vi "log analysis_gps.vi"() -> ()   [LabVIEW 2018] (continued)
7.8801,22.3000,0.1011,-0.2963,-0.0025,0.185692893,-0.737548130,275.721839304,0.4376,0.2941,0.5694,0.1127,0.0923,0.0781,0.0965,0.1014,4.9971,0f000001,0*33922ff8\n\t", "DUALANTENNAHEADINGA,USB3,0,50.0,FINESTEERING,2107,283447.000,02000000,d426,15824;INSUFFICIENT_OBS,NONE,-1.000000000,0.000000000,0.000000000,0.0,0.000000000,0.000000000,\"631T\",11,4,4,3,04,00,20,03*3318e43a\n\t", "DUALANTENNAHEADINGA,USB3,0,51.5,FINESTEERING,2107,283448.500,02000000,d426,15824;INSUFFICIENT_OBS,NONE,-1.000000000,0.000000000,0.000000000,0.0,0.000000000,0.000000000,\"631T\",14,4,4,3,04,00,20,03*e9e47ab5\n\t", "DUALANTENNAHEADINGA,USB3,0,51.5,FINESTEERING,2107,283449.000,02000000,d426,15824;INSUFFICIENT_OBS,NONE,-1.000000000,0.000000000,0.000000000,0.0,0.000000000,0.000000000,\"631T\",12,4,4,3,04,00,20,03*cef36426\n\t", "DUALANTENNAHEADINGA,USB3,0,49.0,FINESTEERING,2107,283450.000,02000000,d426,15824;INSUFFICIENT_OBS,NONE,-1.000000000,0.000000000,0.000000000,0.0,0.000000000,0.000000000,\"631T\",14,4,4,3,04,00,20,03*09d68f9b\n\t", "DUALANTENNAHEADINGA,USB3,0,49.0,FINESTEERING,2107,283450.500,02000000,d426,15824;INSUFFICIENT_OBS,NONE,-1.000000000,0.000000000,0.000000000,0.0,0.000000000,0.000000000,\"631T\",12,4,4,3,04,00,20,03*431995d1\n\t", "DUALANTENNAHEADINGA,USB3,0,49.0,FINESTEERING,2107,283451.000,02000000,d426,15824;INSUFFICIENT_OBS,NONE,-1.000000000,0.000000000,0.000000000,0.0,0.000000000,0.000000000,\"631T\",12,4,4,3,04,00,20,03*f9d28051\n\t", "DUALANTENNAHEADINGA,USB3,0,44.5,FINESTEERING,2107,283451.500,02000000,d426,15824;INSUFFICIENT_OBS,NONE,-1.000000000,0.000000000,0.000000000,0.0,0.000000000,0.000000000,\"631T\",14,4,4,3,04,00,20,03*5c854f00\n\t", "DUALANTENNAHEADINGA,USB3,0,44.5,FINESTEERING,2107,283452.000,02000000,d426,15824;INSUFFICIENT_OBS,NONE,-1.000000000,0.000000000,0.000000000,0.0,0.000000000,0.000000000,\"631T\",14,4,4,3,04,00,20,03*3dfe5332\n\t", "DUALANTENNAHEADINGA,USB3,0,49.0,FINESTEERING,2107,283452.500,02000000,d426,15824;INSUFFICIENT_OBS,NONE,-1.000000000,0.000000000,0.000000000,0.0,0.000000000,0.000000000,\"631T\",12,4,4,3,04,00,20,03*98a99c63\n\t", "DUALANTENNAHEADINGA,USB3,0,49.0,FINESTEERING,2107,283453.000,02000000,d426,15824;INSUFFICIENT_OBS,NONE,-1.000000000,0.000000000,0.000000000,0.0,0.000000000,0.000000000,\"631T\",10,4,4,3,04,00,20,03*56d68f12\n\t", "DUALANTENNAHEADINGA,USB3,0,50.0,FINESTEERING,2107,283453.500,02000000,d426,15824;INSUFFICIENT_OBS,NONE,-1.000000000,0.000000000,0.000000000,0.0,0.000000000,0.000000000,\"631T\",9,4,4,3,04,00,20,02*71c65a10\n\t", "DUALANTENNAHEADINGA,USB3,0,50.0,FINESTEERING,2107,283454.000,02000000,d426,15824;INSUFFICIENT_OBS,NONE,-1.000000000,0.000000000,0.000000000,0.0,0.000000000,0.000000000,\"631T\",10,4,4,3,04,00,20,03*adf0db7d\n\t", "DUALANTENNAHEADINGA,USB3,0,53.5,FINESTEERING,2107,283454.500,02000000,d426,15824;INSUFFICIENT_OBS,NONE,-1.000000000,0.000000000,0.000000000,0.0,0.000000000,0.000000000,\"631T\",10,4,4,3,04,00,20,03*83545704\n\t", "DUALANTENNAHEADINGA,USB3,0,53.5,FINESTEERING,2107,283455.000,02000000,d426,15824;INSUFFICIENT_OBS,NONE,-1.000000000,0.000000000,0.000000000,0.0,0.000000000,0.000000000,\"631T\",10,4,4,3,04,00,20,03*399f4284\n\t", "DUALANTENNAHEADINGA,USB3,0,53.0,FINESTEERING,2107,283455.500,02000000,d426,15824;INSUFFICIENT_OBS,NONE,-1.000000000,0.000000000,0.000000000,0.0,0.000000000,0.000000000,\"631T\",10,4,4,3,04,00,20,03*bbf6b511\n\t", "DUALANTENNAHEADINGA,USB3,0,53.0,FINESTEERING,2107,283456.000,02000000,d426,15824;INSUFFICIENT_OBS,NONE,-1.000000000,0.000000000,0.000000000,0.0,0.000000000,0.000000000,\"631T\",10,4,4,3,04,00,20,03*da8da923\n\t", "DUALANTENNAHEADINGA,USB3,0,50.5,FINESTEERING,2107,283456.500,02000000,d426,15824;INSUFFICIENT_OBS,NONE,-1.000000000,0.000000000,0.000000000,0.0,0.000000000,0.000000000,\"631T\",10,4,4,3,04,00,20,03*f429255a\n\t", "DUALANTENNAHEADINGA,USB3,0,50.5,FINESTEERING,2107,283457.000,02000000,d426,15824;INSUFFICIENT_OBS,NONE,-1.000000000,0.000000000,0.000000000,0.0,0.000000000,0.000000000,\"631T\",11,4,4,3,04,00,20,03*9900b082\n\t", "DUALANTENNAHEADINGA,USB3,0,52.0,FINESTEERING,2107,283457.500,02000000,d426,15824;INSUFFICIENT_OBS,NONE,-1.000000000,0.000000000,0.000000000,0.0,0.000000000,0.000000000,\"631T\",11,4,4,3,04,00,20,03*d3e0ea5f\n\t", "DUALANTENNAHEADINGA,USB3,0,52.0,FINESTEERING,2107,283458.000,02000000,d426,15824;INSUFFICIENT_OBS,NONE,-1.000000000,0.000000000,0.000000000,0.0,0.000000000,0.000000000,\"631T\",12,4,4,3,04,00,20,02*d2f97f3d\n\t", "INSPVAXA,USB3,0,50.0,FINESTEERING,2107,283458.550,02000000,471d,15824;INS_ALIGNMENT_COMPLETE,INS_RTKFIXED,37.37123761110,126.72265482999,7.8240,22.3000,0.0859,-0.2308,-0.0155,0.304728357,-0.212159203,274.715146909,0.4465,0.2951,0.5711,0.1136,0.0925,0.0781,0.0966,0.1016,5.0109,0f000001,0*14308c9c\n\t", "INSPVAXA,USB3,0,50.0,FINESTEERING,2107,283459.050,02000000,471d,15824;INS_ALIGNMENT_COMPLETE,INS_RTKFIXED,37.37123780985,126.72265328103,7.8227,22.3000,0.0882,-0.3585,-0.0269,0.289946645,-0.080144409,275.013875175,0.4463,0.2950,0.5710,0.1135,0.0925,0.0781,0.0966,0.1016,5.0117,0f000001,0*9875c775\n\t", "INSPVAXA,USB3,0,50.5,FINESTEERING,2107,283459.550,02000000,471d,15824;INS_ALIGNMENT_COMPLETE,INS_RTKFIXED,37.37123799841,126.72265173838,7.8223,22.3000,0.0838,-0.2861,-0.0112,0.173844892,-0.010609871,275.281152331,0.4463,0.2950,0.5710,0.1135,0.0925,0.0781,0.0966,0.1016,5.0117,0f000001,0*d5666360\n\t", "INSPVAXA,USB3,0,50.5,FINESTEERING,2107,283460.050,02000000,471d,15824;INS_ALIGNMENT_COMPLETE,INS_RTKFIXED,37.37123822343,126.72265007400,7.8217,22.3000,0.0923,-0.2835,-0.0262,0.253668906,0.084108634,275.465582577,0.4457,0.2949,0.5709,0.1137,0.0925,0.0781,0.0966,0.1016,5.0129,0f000001,0*4b6161dc\n\t", "INSPVAXA,USB3,0,51.5,FINESTEERING,2107,283460.550,02000000,471d,15824;INS_ALIGNMENT_COMPLETE,INS_RTKFIXED,37.37123844435,126.72264849525,7.8205,22.3000,0.0984,-0.3080,-0.0293,0.364026369,0.239403799,275.671224814,0.4457,0.2949,0.5709,0.1137,0.0925,0.0781,0.0966,0.1016,5.0129,0f000001,0*2bf0cdc4\n\t", "DUALANTENNAHEADINGA,USB3,0,51.5,FINESTEERING,2107,283461.000,02000000,d426,15824;INSUFFICIENT_OBS,NONE,-1.000000000,0.000000000,0.000000000,0.0,0.000000000,0.000000000,\"631T\",13,4,4,3,04,00,20,03*e487ac9d\n\t", "INSPVAXA,USB3,0,47.5,FINESTEERING,2107,283461.550,02000000,471d,15824;INS_ALIGNMENT_COMPLETE,INS_RTKFIXED,37.37123893716,126.72264534248,7.8162,22.3000,0.0985,-0.2963,-0.0141,0.697862948,0.169461107,276.143360178,0.4456,0.2948,0.5708,0.1136,0.0924,0.0781,0.0966,0.1015,5.0137,0f000001,0*a30b3e45\n\t", "INSPVAXA,USB3,0,43.5,FINESTEERING,2107,283462.550,02000000,471d,15824;INS_ALIGNMENT_COMPLETE,INS_RTKFIXED,37.37123942098,126.72264211433,7.8134,22.3000,0.0929,-0.3127,-0.0203,0.398142005,-0.231454144,276.636876132,0.4454,0.2949,0.5708,0.1135,0.0925,0.0781,0.0966,0.1015,5.0146,0f000001,0*24e4ed99\n\t", "INSPVAXA,USB3,0,43.5,FINESTEERING,2107,283463.050,02000000,471d,15824;INS_ALIGNMENT_COMPLETE,INS_RTKFIXED,37.37123965098,126.72264063011,7.8119,22.3000,0.0776,-0.1820,-0.0220,0.127573925,-0.349335206,276.957400381,0.4448,0.2950,0.5707,0.1136,0.0925,0.0781,0.0966,0.1015,5.0158,0f000001,0*86cff0c5\n\t", "INSPVAXA,USB3,0,50.0,FINESTEERING,2107,283463.550,02000000,471d,15824;INS_ALIGNMENT_COMPLETE,INS_RTKFIXED,37.37123983702,126.72263968205,7.8117,22.3000,0.1160,-0.4339,-0.0234,0.042320213,-0.166110227,277.135399170,0.4448,0.2950,0.5707,0.1136,0.0925,0.0781,0.0966,0.1015,5.0158,0f000001,0*a9cde56f\n\t", "INSPVAXA,USB3,0,50.5,FINESTEERING,2107,283464.550,02000000,471d,15824;INS_ALIGNMENT_COMPLETE,INS_RTKFIXED,37.37124035890,126.72263654398,7.8101,22.3000,0.0978,-0.3247,-0.0269,0.153067823,0.062690713,277.456657188,0.4447,0.2949,0.5707,0.1135,0.0925,0.0781,0.0966,0.1015,5.0168,0f000001,0*e25a65bd\n\t", "INSPVAXA,USB3,0,47.5,FINESTEERING,2107,283465.550,02008000,471d,15824;INS_ALIGNMENT_COMPLETE,INS_RTKFIXED,37.37124087816,126.72263323359,7.8095,22.3000,0.1048,-0.3207,-0.0188,-0.139743326,-0.216469066,277.649451326,0.4444,0.2948,0.5707,0.1135,0.0925,0.0781,0.0966,0.1015,5.0179,0f000001,0*3b3a13db\n\t", "INSPVAXA,USB3,0,47.0,FINESTEERING,2107,283466.050,02008000,471d,15824;INS_ALIGNMENT_COMPLETE,INS_RTKFIXED,37.37124115647,126.72263161557,7.8102,22.3000,0.1038,-0.3165,-0.0156,-0.037052070,-0.429278496,277.644852410,0.4437,0.2948,0.5706,0.1136,0.0925,0.0781,0.0966,0.1015,5.0190,0f000001,0*71415a25\n\t", "INSPVAXA,USB3,0,46.5,FINESTEERING,2107,283467.050,02008000,471d,15824;INS_ALIGNMENT_COMPLETE,INS_RTKFIXED,37.37124175185,126.72262828673,7.8114,22.3000,0.1144,-0.3107,-0.0235,0.189502130,-0.846127382,277.724037257,0.4428,0.2947,0.5707,0.1137,0.0925,0.0781,0.0965,0.1015,5.0203,0f000001,0*123a4309\n\t", "INSPVAXA,USB3,0,46.5,FINESTEERING,2107,283467.550,02008000,471d,15824;INS_ALIGNMENT_COMPLETE,INS_RTKFIXED,37.37124201534,126.72262669568,7.8140,22.3000,0.1123,-0.3073,-0.0295,0.009270111,-0.651900427,277.586297393,0.4428,0.2947,0.5707,0.1137,0.0925,0.0781,0.0965,0.1015,5.0203,0f000001,0*fbe18a0e\n\t", "INSPVAXA,USB3,0,46.5,FINESTEERING,2107,283468.050,02008000,471d,15824;INS_ALIGNMENT_COMPLETE,INS_RTKFIXED,37.37124222504,126.72262566051,7.8172,22.3000,0.1108,-0.3362,-0.0087,-0.107061693,-0.300479495,277.280043662,0.4419,0.2947,0.5706,0.1134,0.0926,0.0781,0.0965,0.1015,5.0216,0f000001,0*e4f8bd3b\n\t", "INSPVAXA,USB3,0,46.5,FINESTEERING,2107,283468.550,02008000,471d,15824;INS_ALIGNMENT_COMPLETE,INS_RTKFIXED,37.37124250886,126.72262396333,7.8186,22.3000,0.0904,-0.2606,-0.0155,0.241398611,-0.239914354,276.982575871,0.4419,0.2947,0.5706,0.1134,0.0926,0.0781,0.0965,0.1015,5.0216,0f000001,0*b84fac19\n\t", "INSPVAXA,USB3,0,46.5,FINESTEERING,2107,283469.050,02008000,471d,15824;INS_ALIGNMENT_COMPLETE,INS_RTKFIXED,37.37124277441,126.72262234556,7.8204,22.3000,0.0912,-0.2797,-0.0071,0.371726808,-0.134537847,276.502900110,0.4420,0.2946,0.5707,0.1134,0.0925,0.0781,0.0965,0.1015,5.0228,0f000001,0*e3b85341\n\t", "INSPVAXA,USB3,0,46.5,FINESTEERING,2107,283469.550,02000000,471d,15824;INS_ALIGNMENT_COMPLETE,INS_RTKFIXED,37.37124299469,126.72262074731,7.8238,22.3000,0.0920,-0.2961,-0.0076,0.268432446,-0.051624377,275.936964776,0.4420,0.2946,0.5707,0.1134,0.0925,0.0781,0.0965,0.1015,5.0228,0f000001,0*2bf39c83\n\t", "INSPVAXA,USB3,0,46.5,FINESTEERING,2107,283470.050,02000000,471d,15824;INS_ALIGNMENT_COMPLETE,INS_RTKFIXED,37.37124320185,126.72261913294,7.8277,22.3000,0.1016,-0.3039,-0.0081,0.097334282,-0.040914824,275.470071577,0.4421,0.2945,0.5705,0.1133,0.0925,0.0781,0.0965,0.1015,5.0240,0f000001,0*fba59bc0\n\t", "INSPVAXA,USB3,0,46.0,FINESTEERING,2107,283470.550,02000000,471d,15824;INS_ALIGNMENT_COMPLETE,INS_RTKFIXED,37.37124338791,126.72261753041,7.8308,22.3000,0.0952,-0.3085,-0.0166,0.133198761,-0.149300004,274.919636182,0.4421,0.2945,0.5705,0.1133,0.0925,0.0781,0.0965,0.1015,5.0240,0f000001,0*42261ade\n\t", "INSPVAXA,USB3,0,46.0,FINESTEERING,2107,283471.050,02000000,471d,15824;INS_ALIGNMENT_COMPLETE,INS_RTKFIXED,37.37124356076,126.72261595668,7.8336,22.3000,0.0792,-0.2815,-0.0153,0.105112248,-0.115677362,274.303120166,0.4420,0.2946,0.5706,0.1132,0.0925,0.0781,0.0964,0.1015,5.0248,0f000001,0*c06838c2\n\t", "INSPVAXA,USB3,0,48.0,FINESTEERING,2107,283471.550,02000000,471d,15824;INS_ALIGNMENT_COMPLETE,INS_RTKFIXED,37.37124371844,126.72261435668,7.8362,22.3000,0.0861,-0.3146,0.0012,0.009847777,-0.154362350,273.837649570,0.4420,0.2946,0.5706,0.1132,0.0925,0.0781,0.0964,0.1015,5.0248,0f000001,0*248758d2\n\t", "INSPVAXA,USB3,0,48.0,FINESTEERING,2107,283472.050,02000000,471d,15824;INS_ALIGNMENT_COMPLETE,INS_RTKFIXED,37.37124388873,126.72261272959,7.8390,22.3000,0.0744,-0.3068,0.0071,0.047718600,-0.362449077,273.522239359,0.4416,0.2945,0.5705,0.1131,0.0924,0.0781,0.0964,0.1014,5.0253,0f000001,0*b034cfcb\n\t", "INSPVAXA,USB3,0,48.5,FINESTEERING,2107,283473.050,02000000,471d,15824;INS_ALIGNMENT_COMPLETE,INS_RTKFIXED,37.37124418423,126.72260986099,7.8423,22.3000,0.0465,-0.2147,-0.0152,-0.064754413,-0.661648789,273.035495694,0.4408,0.2944,0.5705,0.1130,0.0925,0.0781,0.0964,0.1014,5.0261,0f000001,0*8452aba9\n\t", "INSPVAXA,USB3,0,49.5,FINESTEERING,2107,283473.550,02000000,471d,15824;INS_ALIGNMENT_COMPLETE,INS_RTKFIXED,37.37124432645,126.72260825595,7.8450,22.3000,0.0577,-0.2717,-0.0116,-0.371304457,-0.586321968,273.022512586,0.4408,0.2944,0.5705,0.1130,0.0925,0.0781,0.0964,0.1014,5.0261,0f000001,0*dc18a2a0\n\t", "INSPVAXA,USB3,0,49.5,FINESTEERING,2107,283474.050,02000000,471d,15824;INS_ALIGNMENT_COMPLETE,INS_RTKFIXED,37.37124450056,126.72260664706,7.8482,22.3000,0.0746,-0.3111,-0.0073,-0.324886266,-0.572903828,273.001550597,0.4404,0.2944,0.5705,0.1132,0.0924,0.0781,0.0964,0.1014,5.0269,0f000001,0*6a9d6035\n\t", "INSPVAXA,USB3,0,47.5,FINESTEERING,2107,283474.550,02000000,471d,15824;INS_ALIGNMENT_COMPLETE,INS_RTKFIXED,37.37124465803,126.72260513334,7.8520,22.3000,0.0754,-0.3176,-0.0107,-0.183521843,-0.419147720,273.001614908,0.4404,0.2944,0.5705,0.1132,0.0924,0.0781,0.0964,0.1014,5.0269,0f000001,0*c3ef68c2\n\t", "INSPVAXA,USB3,0,47.5,FINESTEERING,2107,283475.050,02000000,471d,15824;INS_ALIGNMENT_COMPLETE,INS_RTKFIXED,37.37124482420,126.72260357530,7.8549,22.3000,0.0753,-0.2803,-0.0146,-0.241068696,-0.296923689,273.106112886,0.4399,0.2945,0.5706,0.1130,0.0924,0.0781,0.0964,0.1014,5.0279,0f000001,0*9f37bee3\n\t", "INSPVAXA,USB3,0,47.5,FINESTEERING,2107,283475.550,02000000,471d,15824;INS_ALIGNMENT_COMPLETE,INS_RTKFIXED,37.37124499067,126.72260199547,7.8565,22.3000,0.0685,-0.2996,-0.0135,-0.434680931,-0.247748012,273.252507934,0.4399,0.2945,0.5706,0.1130,0.0924,0.0781,0.0964,0.1014,5.0279,0f000001,0*f6dcb523\n\t", "INSPVAXA,USB3,0,47.5,FINESTEERING,2107,283476.050,02000000,471d,15824;INS_ALIGNMENT_COMPLETE,INS_RTKFIXED,37.37124517702,126.72260043999,7.8594,22.3000,0.0731,-0.2995,-0.0095,-0.441036624,-0.242977977,273.321134070,0.4399,0.2945,0.5707,0.1130,0.0924,0.0781,0.0964,0.1014,5.0290,0f000001,0*df4d40ec\n\t", "INSPVAXA,USB3,0,50.0,FINESTEERING,2107,283476.550,02000000,471d,15824;INS_ALIGNMENT_COMPLETE,INS_RTKFIXED,37.37124535364,126.72259887050,7.8616,22.3000,0.0731,-0.2996,-0.0100,-0.412710306,-0.285107992,273.399842482,0.4399,0.2945,0.5707,0.1130,0.0924,0.0781,0.0964,0.1014,5.0290,0f000001,0*4ef28dbb\n\t", "INSPVAXA,USB3,0,51.0,FINESTEERING,2107,283477.550,02000000,471d,15824;INS_ALIGNMENT_COMPLETE,INS_RTKFIXED,37.37124569782,126.72259576074,7.8655,22.3000,0.0695,-0.3003,-0.0075,-0.469235251,-0.455743841,273.579264680,0.4397,0.2945,0.5707,0.1130,0.0924,0.0781,0.0964,0.1014,5.0303,0f000001,0*db0f6a2f\n\t", "INSPVAXA,USB3,0,51.0,FINESTEERING,2107,283478.050,02000000,471d,15824;INS_ALIGNMENT_COMPLETE,INS_RTKFIXED,37.37124587328,126.72259421546,7.8690,22.3000,0.0786,-0.2811,0.0029,-0.458800403,-0.268524381,273.658587255,0.4407,0.2947,0.5709,0.1132,0.0924,0.0781,0.0964,0.1014,5.0316,0f000001,0*f403e502\n\t", "INSPVAXA,USB3,0,51.0,FINESTEERING,2107,283478.550,02000000,471d,15824;INS_ALIGNMENT_COMPLETE,INS_RTKFIXED,37.37124604525,126.72259266223,7.8723,22.3000,0.0753,-0.2945,0.0030,-0.462352826,-0.136958884,273.744107735,0.4407,0.2947,0.5709,0.1132,0.0924,0.0781,0.0964,0.1014,5.0316,0f000001,0*3bf5fab5\n\t", "INSPVAXA,USB3,0,51.0,FINESTEERING,2107,283479.050,02000000,471d,15824;INS_ALIGNMENT_COMPLETE,INS_RTKFIXED,37.37124622444,126.72259108516,7.8745,22.3000,0.0782,-0.2955,0.0000,-0.529822830,0.178727443,273.870016111,0.4415,0.2947,0.5709,0.1133,0.0924,0.0781,0.0964,0.1014,5.0329,0f000001,0*0db861ca\n\t", "INSPVAXA,USB3,0,51.0,FINESTEERING,2107,283479.550,02000000,471d,15824;INS_ALIGNMENT_COMPLETE,INS_RTKFIXED,37.37124640170,126.72258950006,7.8775,22.3000,0.0805,-0.3037,0.0007,-0.509921072,0.195230583,273.949901234,0.4415,0.2947,0.5709,0.1133,0.0924,0.0781,0.0964,0.1014,5.0329,0f000001,0*077866b6\n\t", "INSPVAXA,USB3,0,51.0,FINESTEERING,2107,283480.050,02000000,471d,15824;INS_ALIGNMENT_COMPLETE,INS_RTKFIXED,37.37124659299,126.72258788570,7.8812,22.3000,0.0832,-0.3022,-0.0023,-0.414591825,-0.152431490,274.036956074,0.4426,0.2949,0.5711,0.1133,0.0924,0.0781,0.0964,0.1014,5.0343,0f000001,0*6e70f737\n\t", "INSPVAXA,USB3,0,50.0,FINESTEERING,2107,283481.550,02000000,471d,15824;INS_ALIGNMENT_COMPLETE,INS_RTKFIXED,37.37124714529,126.72258299767,7.8939,22.3000,0.0873,-0.3069,-0.0133,-0.586135229,-0.604059291,274.319909589,0.4441,0.2951,0.5712,0.1135,0.0925,0.0781,0.0964,0.1015,5.0357,0f000001,0*8645286f\n\t", "INSPVAXA,USB3,0,51.0,FINESTEERING,2107,283482.550,02000000,471d,15824;INS_ALIGNMENT_COMPLETE,INS_RTKFIXED,37.37124752948,126.72258005871,7.9006,22.3000,0.0687,-0.3152,0.0109,-0.135978920,-0.255823048,274.401094363,0.4449,0.2953,0.5713,0.1139,0.0925,0.0782,0.0964,0.1015,5.0373,0f000001,0*5cec8015\n\t", "INSPVAXA,USB3,0,51.5,FINESTEERING,2107,283484.050,02000000,471d,15824;INS_ALIGNMENT_COMPLETE,INS_RTKFIXED,37.37124809880,126.72257534904,7.9142,22.3000,0.0705,-0.2771,0.0043,-0.387988149,0.243310051,274.386615848,0.4464,0.2955,0.5716,0.1138,0.0925,0.0782,0.0964,0.1015,5.0399,0f000001,0*6b4a4f7e\n\t", "INSPVAXA,USB3,0,53.5,FINESTEERING,2107,283485.050,02000000,471d,15824;INS_ALIGNMENT_COMPLETE,INS_RTKFIXED,37.37124849221,126.72257218238,7.9219,22.3000,0.0806,-0.2954,-0.0022,-0.251628518,0.390951997,274.060594650,0.4471,0.2956,0.5717,0.1137,0.0925,0.0782,0.0964,0.1014,5.0410,0f000001,0*78d5c28f\n\t", "INSPVAXA,USB3,0,51.0,FINESTEERING,2107,283485.550,02000000,471d,15824;INS_ALIGNMENT_COMPLETE,INS_RTKFIXED,37.37124867338,126.72257057546,7.9253,22.3000,0.0807,-0.2982,0.0046,-0.297126660,0.143555432,273.789468415,0.4471,0.2956,0.5717,0.1137,0.0925,0.0782,0.0964,0.1014,5.0410,0f000001,0*c848650b\n\t", "INSPVAXA,USB3,0,46.0,FINESTEERING,2107,283486.050,02000000,471d,15824;INS_ALIGNMENT_COMPLETE,INS_RTKFIXED,37.37124886174,126.72256897160,7.9281,22.3000,0.0774,-0.2942,-0.0013,-0.283569757,0.106976902,273.570280777,0.4473,0.2956,0.5718,0.1136,0.0925,0.0782,0.0964,0.1014,5.0421,0f000001,0*a5ad5170\n\t", "INSPVAXA,USB3,0,48.0,FINESTEERING,2107,283487.550,02000000,471d,15824;INS_ALIGNMENT_COMPLETE,INS_RTKFIXED,37.37124935038,126.72256433363,7.9396,22.3000,0.0684,-0.2764,-0.0073,-0.272700392,-0.138830686,272.596264652,0.4472,0.2956,0.5720,0.1137,0.0925,0.0782,0.0964,0.1014,5.0432,0f000001,0*7a2c3ea8\n\t", "INSPVAXA,USB3,0,48.0,FINESTEERING,2107,283488.050,02000000,471d,15824;INS_ALIGNMENT_COMPLETE,INS_RTKFIXED,37.37124950186,126.72256271851,7.9401,22.3000,0.0702,-0.2701,-0.0123,-0.306984619,-0.156481327,272.240352171,0.4472,0.2957,0.5722,0.1136,0.0925,0.0782,0.0964,0.1014,5.0443,0f000001,0*50a165ff\n\t", "INSPVAXA,USB3,0,48.5,FINESTEERING,2107,283488.550,02000000,471d,15824;INS_ALIGNMENT_COMPLETE,INS_RTKFIXED,37.37124963696,126.72256112600,7.9399,22.3000,0.0634,-0.2924,-0.0061,-0.348692985,-0.211479337,271.855613875,0.4472,0.2957,0.5722,0.1136,0.0925,0.0782,0.0964,0.1014,5.0443,0f000001,0*ed71010c\n\t", "INSPVAXA,USB3,0,49.0,FINESTEERING,2107,283489.550,02000000,471d,15824;INS_ALIGNMENT_COMPLETE,INS_RTKFIXED,37.37124992844,126.72255789438,7.9412,22.3000,0.0625,-0.2932,0.0092,-0.217423535,-0.472312164,271.147208708,0.4467,0.2958,0.5722,0.1138,0.0925,0.0782,0.0964,0.1014,5.0457,0f000001,0*6d85d9a8\n\t", "INSPVAXA,USB3,0,49.0,FINESTEERING,2107,283490.050,02000000,471d,15824;INS_ALIGNMENT_COMPLETE,INS_RTKFIXED,37.37125008339,126.72255625341,7.9419,22.3000,0.0636,-0.2955,0.0152,0.008734422,-0.613623948,270.920387351,0.4456,0.2958,0.5721,0.1138,0.0926,0.0782,0.0964,0.1014,5.0473,0f000001,0*aa76f15f\n\t", "INSPVAXA,USB3,0,52.5,FINESTEERING,2107,283490.550,02000000,471d,15824;INS_ALIGNMENT_COMPLETE,INS_RTKFIXED,37.37125019673,126.72255461280,7.9407,22.3000,0.0735,-0.3073,0.0114,-0.028034352,-0.928675652,270.685326293,0.4456,0.2958,0.5721,0.1138,0.0926,0.0782,0.0964,0.1014,5.0473,0f000001,0*cd41eb0e\n\t", "INSPVAXA,USB3,0,49.5,FINESTEERING,2107,283500.050,02000000,471d,15824;INS_ALIGNMENT_COMPLETE,INS_RTKFIXED,37.37125208894,126.72252418884,7.9323,22.3000,0.0457,-0.3130,0.0162,0.019884592,-0.737230354,268.941103131,0.4422,0.2953,0.5719,0.1133,0.0925,0.0782,0.0964,0.1015,5.0570,0f000001,0*24f2188e\n\t", "INSPVAXA,USB3,0,48.5,FINESTEERING,2107,283508.100,02000000,471d,15824;INS_ALIGNMENT_COMPLETE,INS_RTKFIXED,37.37125276901,126.72249960907,7.9453,22.3000,0.0373,-0.2902,0.0053,-0.191217202,-0.027683345,268.229043523,0.4412,0.2949,0.5722,0.1131,0.0925,0.0782,0.0964,0.1013,5.0646,0f000001,0*8b85f82b\n\t", "INSPVAXA,USB3,0,51.0,FINESTEERING,2107,283509.100,02000000,471d,15824;INS_ALIGNMENT_COMPLETE,INS_RTKFIXED,37.37125284410,126.72249644466,7.9470,22.3000,0.0401,-0.2879,-0.0045,-0.106806668,-0.162103067,268.404823616,0.4419,0.2950,0.5723,0.1130,0.0925,0.0782,0.0964,0.1013,5.0643,0f000001,0*7bfc8e45\n\t", "INSPVAXA,USB3,0,49.5,FINESTEERING,2107,283511.100,02000000,471d,15824;INS_ALIGNMENT_COMPLETE,INS_RTKFIXED,37.37125297857,126.72249062368,7.9478,22.3000,0.0268,-0.2671,0.0078,-0.192910717,-0.348782343,268.576521671,0.4435,0.2952,0.5725,0.1132,0.0925,0.0782,0.0964,0.1012,5.0632,0f000001,0*b468220b\n\t", "INSPVAXA,USB3,0,46.5,FINESTEERING,2107,283512.100,02000000,471d,15824;INS_ALIGNMENT_COMPLETE,INS_RTKFIXED,37.37125304820,126.72248734658,7.9477,22.3000,0.0144,-0.2984,0.0121,-0.146751568,-0.096737224,268.816557460,0.4452,0.2954,0.5727,0.1133,0.0925,0.0782,0.0964,0.1013,5.0625,0f000001,0*292499ae\n\t", "INSPVAXA,USB3,0,46.5,FINESTEERING,2107,283512.600,02000000,471d,15824;INS_ALIGNMENT_COMPLETE,INS_RTKFIXED,37.37125307400,126.72248575305,7.9480,22.3000,0.0122,-0.2749,0.0049,-0.358672753,0.036676838,268.917809450,0.4452,0.2954,0.5727,0.1133,0.0925,0.0782,0.0964,0.1013,5.0625,0f000001,0*09269caa\n\t", "INSPVAXA,USB3,0,46.0,FINESTEERING,2107,283516.100,02000000,471d,15824;INS_ALIGNMENT_COMPLETE,INS_RTKFIXED,37.37125347923,126.72247506393,7.9472,22.3000,0.0170,-0.3545,-0.0054,-0.698217493,-0.526151709,269.397858351,0.4451,0.2957,0.5732,0.1136,0.0925,0.0782,0.0963,0.1013,5.0659,0f000001,0*b20fee82\n\t", "INSPVAXA,USB3,0,52.0,FINESTEERING,2107,283517.100,02000000,471d,15824;INS_ALIGNMENT_COMPLETE,INS_RTKFIXED,37.37125363028,126.72247167466,7.9449,22.3000,0.0243,-0.3135,0.0010,-0.686347073,-0.797841284,269.600362862,0.4443,0.2956,0.5732,0.1135,0.0925,0.0782,0.0963,0.1013,5.0669,0f000001,0*80e32c69\n\t", "INSPVAXA,USB3,0,49.0,FINESTEERING,2107,283518.600,02000000,471d,15824;INS_ALIGNMENT_COMPLETE,INS_RTKFIXED,37.37125389857,126.72246679519,7.9445,22.3000,0.0331,-0.3036,0.0138,-0.450567847,-0.447424519,269.738401914,0.4438,0.2956,0.5732,0.1134,0.0925,0.0782,0.0963,0.1013,5.0679,0f000001,0*e0521a7f\n\t", "INSPVAXA,USB3,0,48.0,FINESTEERING,2107,283520.100,02000000,471d,15824;INS_ALIGNMENT_COMPLETE,INS_RTKFIXED,37.37125419691,126.72246226393,7.9458,22.3000,0.0272,-0.1971,0.0083,-0.453121577,-0.197375891,269.782721447,0.4440,0.2956,0.5733,0.1137,0.0925,0.0782,0.0963,0.1013,5.0706,0f000001,0*56a37df9\n\t", "INSPVAXA,USB3,0,51.0,FINESTEERING,2107,283520.600,02000000,471d,15824;INS_ALIGNMENT_COMPLETE,INS_RTKFIXED,37.37125430556,126.72246059927,7.9481,22.3000,0.0288,-0.2781,0.0031,-0.463416060,-0.290924424,269.736679663,0.4440,0.2956,0.5733,0.1137,0.0925,0.0782,0.0963,0.1013,5.0706,0f000001,0*484206e1\n\t", "INSPVAXA,USB3,0,50.0,FINESTEERING,2107,283522.100,02000000,471d,15824;INS_ALIGNMENT_COMPLETE,INS_RTKFIXED,37.37125461142,126.72245575598,7.9554,22.3000,0.0322,-0.2902,-0.0060,-0.575699494,-0.254956238,269.403721782,0.4439,0.2957,0.5734,0.1134,0.0925,0.0782,0.0963,0.1013,5.0736,0f000001,0*4d3ff4ec\n\t", "INSPVAXA,USB3,0,50.0,FINESTEERING,2107,283522.600,02000000,471d,15824;INS_ALIGNMENT_COMPLETE,INS_RTKFIXED,37.37125471396,126.72245415918,7.9561,22.3000,0.0355,-0.2916,-0.0127,-0.527584053,-0.253715800,269.126606548,0.4439,0.2957,0.5734,0.1134,0.0925,0.0782,0.0963,0.1013,5.0736,0f000001,0*ec5fc995\n\t", "INSPVAXA,USB3,0,48.5,FINESTEERING,2107,283523.100,02000000,471d,15824;INS_ALIGNMENT_COMPLETE,INS_RTKFIXED,37.37125482190,126.72245252510,7.9566,22.3000,0.0302,-0.2961,-0.0010,-0.338922460,-0.418464715,268.895183147,0.4433,0.2957,0.5734,0.1134,0.0926,0.0782,0.0963,0.1013,5.0752,0f000001,0*1d6fb429\n\t", "INSPVAXA,USB3,0,48.5,FINESTEERING,2107,283523.600,02000000,471d,15824;INS_ALIGNMENT_COMPLETE,INS_RTKFIXED,37.37125490537,126.72245090226,7.9573,22.3000,0.0299,-0.3022,0.0033,-0.516635552,-0.400593547,268.699996239,0.4433,0.2957,0.5734,0.1134,0.0926,0.0782,0.0963,0.1013,5.0752,0f000001,0*027b4151\n\t", "INSPVAXA,USB3,0,49.5,FINESTEERING,2107,283524.100,02000000,471d,15824;INS_ALIGNMENT_COMPLETE,INS_RTKFIXED,37.37125498193,126.72244929891,7.9584,22.3000,0.0403,-0.2922,0.0032,-0.646627486,-0.365479151,268.410156940,0.4428,0.2959,0.5733,0.1133,0.0925,0.0782,0.0963,0.1013,5.0766,0f000001,0*7811970f\n\t", "INSPVAXA,USB3,0,47.5,FINESTEERING,2107,283525.600,02000000,471d,15824;INS_ALIGNMENT_COMPLETE,INS_RTKFIXED,37.37125519906,126.72244452104,7.9610,22.3000,0.0264,-0.2896,0.0115,-0.459568698,-0.292533166,267.670803857,0.4424,0.2958,0.5732,0.1133,0.0925,0.0782,0.0963,0.1013,5.0781,0f000001,0*17724b4e\n\t", "INSPVAXA,USB3,0,47.0,FINESTEERING,2107,283526.100,02008000,471d,15824;INS_ALIGNMENT_COMPLETE,INS_RTKFIXED,37.37125524446,126.72244292133,7.9621,22.3000,0.0343,-0.2757,0.0102,-0.752609295,-0.423876797,267.522844293,0.4423,0.2959,0.5731,0.1133,0.0925,0.0782,0.0963,0.1013,5.0795,0f000001,0*e02a1c85\n\t", "INSPVAXA,USB3,0,47.0,FINESTEERING,2107,283527.100,02008000,471d,15824;INS_ALIGNMENT_COMPLETE,INS_RTKFIXED,37.37125535577,126.72243973319,7.9657,22.3000,0.0385,-0.2807,-0.0002,-0.916031014,-0.466994988,267.419817945,0.4418,0.2957,0.5731,0.1132,0.0925,0.0782,0.0963,0.1013,5.0811,0f000001,0*de1342cb\n\t", "INSPVAXA,USB3,0,48.0,FINESTEERING,2107,283527.600,02008000,471d,15824;INS_ALIGNMENT_COMPLETE,INS_RTKFIXED,37.37125539878,126.72243810634,7.9658,22.3000,0.0326,-0.2757,-0.0036,-1.071635503,-0.660283197,267.417863682,0.4418,0.2957,0.5731,0.1132,0.0925,0.0782,0.0963,0.1013,5.0811,0f000001,0*715093d1\n\t", "INSPVAXA,USB3,0,46.5,FINESTEERING,2107,283528.100,02008000,471d,15824;INS_ALIGNMENT_COMPLETE,INS_RTKFIXED,37.37125544077,126.72243647488,7.9658,22.3000,0.0284,-0.2919,-0.0061,-1.262244823,-0.886371740,267.477769914,0.4412,0.2955,0.5730,0.1131,0.0925,0.0782,0.0963,0.1013,5.0826,0f000001,0*a5d2d267\n\t", "INSPVAXA,USB3,0,51.5,FINESTEERING,2107,283529.100,02008000,471d,15824;INS_ALIGNMENT_COMPLETE,INS_RTKFIXED,37.37125551038,126.72243332814,7.9661,22.3000,0.0230,-0.2496,0.0003,-1.593217414,-1.364879356,267.511520433,0.4406,0.2953,0.5729,0.1132,0.0926,0.0782,0.0963,0.1012,5.0841,0f000001,0*c5d25f23\n\t", "INSPVAXA,USB3,0,51.5,FINESTEERING,2107,283529.600,02008000,471d,15824;INS_ALIGNMENT_COMPLETE,INS_RTKFIXED,37.37125553545,126.72243179074,7.9678,22.3000,0.0177,-0.3268,0.0196,-1.900322132,-1.296600351,267.646844528,0.4406,0.2953,0.5729,0.1132,0.0926,0.0782,0.0963,0.1012,5.0841,0f000001,0*bf0a8b51\n\t", "INSPVAXA,USB3,0,51.0,FINESTEERING,2107,283530.100,02008000,471d,15824;INS_ALIGNMENT_COMPLETE,INS_RTKFIXED,37.37125556979,126.72243022543,7.9689,22.3000,0.0347,-0.2712,0.0165,-2.106253221,-1.191638715,267.711415615,0.4397,0.2950,0.5729,0.1130,0.0929,0.0782,0.0963,0.1012,5.0852,0f000001,0*30fd5459\n\t", "INSPVAXA,USB3,0,51.0,FINESTEERING,2107,283530.600,02000000,471d,15824;INS_ALIGNMENT_COMPLETE,INS_RTKFIXED,37.37125561825,126.72242855799,7.9691,22.3000,0.0407,-0.2688,0.0120,-2.213736166,-1.038882938,267.844151397,0.4397,0.2950,0.5729,0.1130,0.0929,0.0782,0.0963,0.1012,5.0852,0f000001,0*ed713259\n\t", "INSPVAXA,USB3,0,43.5,FINESTEERING,2107,283531.100,02000000,471d,15824;INS_ALIGNMENT_COMPLETE,INS_RTKFIXED,37.37125567803,126.72242699713,7.9701,22.3000,0.0384,-0.2967,0.0169,-2.258821559,-0.728124735,267.962573337,0.4398,0.2947,0.5728,0.1130,0.0928,0.0782,0.0963,0.1012,5.0855,0f000001,0*96bde39a\n\t", "INSPVAXA,USB3,0,43.5,FINESTEERING,2107,283531.600,02000000,471d,15824;INS_ALIGNMENT_COMPLETE,INS_RTKFIXED,37.37125573053,126.72242543109,7.9712,22.3000,0.0393,-0.2946,0.0161,-2.393557008,-0.508805819,268.092577363,0.4398,0.2947,0.5728,0.1130,0.0928,0.0782,0.0963,0.1012,5.0855,0f000001,0*fb176aea\n\t", "INSPVAXA,USB3,0,46.5,FINESTEERING,2107,283532.600,02000000,471d,15824;INS_ALIGNMENT_COMPLETE,INS_RTKFIXED,37.37125585668,126.72242215627,7.9725,22.3000,0.0380,-0.3002,0.0167,-2.444436463,-0.411927002,268.408506598,0.4408,0.2948,0.5728,0.1133,0.0928,0.0782,0.0963,0.1013,5.0851,0f000001,0*752f38e5\n\t", "INSPVAXA,USB3,0,46.5,FINESTEERING,2107,283533.100,02000000,471d,15824;INS_ALIGNMENT_COMPLETE,INS_RTKFIXED,37.37125592571,126.72242055610,7.9738,22.3000,0.0424,-0.2920,0.0172,-2.420399044,-0.549310631,268.532317727,0.4414,0.2948,0.5728,0.1132,0.0926,0.0782,0.0963,0.1012,5.0840,0f000001,0*330bd1f6\n\t", "INSPVAXA,USB3,0,49.5,FINESTEERING,2107,283533.600,02000000,471d,15824;INS_ALIGNMENT_COMPLETE,INS_RTKFIXED,37.37125599617,126.72241909319,7.9758,22.3000,0.0239,-0.2932,0.0057,-2.389135000,-0.690009705,268.630043000,0.4414,0.2948,0.5728,0.1132,0.0926,0.0782,0.0963,0.1012,5.0840,0f000001,0*946e4f45\n\t", "INSPVAXA,USB3,0,46.5,FINESTEERING,2107,283534.100,02000000,471d,15824;INS_ALIGNMENT_COMPLETE,INS_RTKFIXED,37.37125606459,126.72241729161,7.9768,22.3000,0.0318,-0.3014,0.0051,-2.433419723,-0.928712698,268.813892776,0.4412,0.2949,0.5728,0.1131,0.0925,0.0782,0.0963,0.1012,5.0833,0f000001,0*8f6d80c9\n\t", "INSPVAXA,USB3,0,46.5,FINESTEERING,2107,283534.600,02000000,471d,15824;INS_ALIGNMENT_COMPLETE,INS_RTKFIXED,37.37125615079,126.72241575292,7.9767,22.3000,0.0422,-0.2723,0.0071,-2.318351029,-0.994572866,268.928791382,0.4412,0.2949,0.5728,0.1131,0.0925,0.0782,0.0963,0.1012,5.0833,0f000001,0*09e2fdbf\n\t", "INSPVAXA,USB3,0,46.5,FINESTEERING,2107,283535.100,02000000,471d,15824;INS_ALIGNMENT_COMPLETE,INS_RTKFIXED,37.37125625866,126.72241406717,7.9767,22.3000,0.0424,-0.2966,-0.0053,-2.021295828,-1.106669357,269.086555595,0.4405,0.2950,0.5729,0.1131,0.0926,0.0782,0.0963,0.1012,5.0840,0f000001,0*6efa0b45\n\t", "INSPVAXA,USB3,0,46.5,FINESTEERING,2107,283535.600,02000000,471d,15824;INS_ALIGNMENT_COMPLETE,INS_RTKFIXED,37.37125636363,126.72241247006,7.9775,22.3000,0.0475,-0.2765,0.0068,-1.865554802,-1.007723760,269.206912297,0.4405,0.2950,0.5729,0.1131,0.0926,0.0782,0.0963,0.1012,5.0840,0f000001,0*0c6af5d6\n\t", "INSPVAXA,USB3,0,47.5,FINESTEERING,2107,283536.100,02000000,471d,15824;INS_ALIGNMENT_COMPLETE,INS_RTKFIXED,37.37125647369,126.72241083113,7.9788,22.3000,0.0521,-0.3007,0.0049,-1.790943231,-0.806222731,269.320889615,0.4398,0.2953,0.5729,0.1129,0.0928,0.0782,0.0963,0.1012,5.0856,0f000001,0*d4e8effb\n\t", "INSPVAXA,USB3,0,47.5,FINESTEERING,2107,283536.600,02000000,471d,15824;INS_ALIGNMENT_COMPLETE,INS_RTKFIXED,37.37125658130,126.72240921238,7.9784,22.3000,0.0588,-0.2967,0.0032,-1.856879731,-0.578836067,269.400871435,0.4398,0.2953,0.5729,0.1129,0.0928,0.0782,0.0963,0.1012,5.0856,0f000001,0*690b56d4\n\t", "INSPVAXA,USB3,0,46.0,FINESTEERING,2107,283537.100,02000000,471d,15824;INS_ALIGNMENT_COMPLETE,INS_RTKFIXED,37.37125671293,126.72240759051,7.9784,22.3000,0.0622,-0.2885,0.0100,-1.691821646,-0.334147317,269.491731881,0.4392,0.2956,0.5729,0.1129,0.0929,0.0782,0.0963,0.1012,5.0866,0f000001,0*9d354d84\n\t", "INSPVAXA,USB3,0,46.0,FINESTEERING,2107,283537.600,02000000,471d,15824;INS_ALIGNMENT_COMPLETE,INS_RTKFIXED,37.37125683698,126.72240594411,7.9786,22.3000,0.0572,-0.2873,0.0166,-1.418143186,-0.126899320,269.581521554,0.4392,0.2956,0.5729,0.1129,0.0929,0.0782,0.0963,0.1012,5.0866,0f000001,0*6d004f4c\n\t", "INSPVAXA,USB3,0,49.0,FINESTEERING,2107,283538.100,02000000,471d,15824;INS_ALIGNMENT_COMPLETE,INS_RTKFIXED,37.37125695995,126.72240477426,7.9799,22.3000,0.0495,-0.1342,0.0227,-1.319474925,-0.166358731,269.556076061,0.4404,0.2961,0.5730,0.1144,0.0933,0.0783,0.0963,0.1012,5.0866,0f000001,0*5c5cf594\n\t", "INSPVAXA,USB3,0,49.0,FINESTEERING,2107,283538.600,02000000,471d,15824;INS_ALIGNMENT_COMPLETE,INS_RTKFIXED,37.37125706097,126.72240298813,7.9830,22.3000,0.0438,-0.2893,0.0273,-1.369512709,-0.160060416,269.600478230,0.4404,0.2961,0.5730,0.1144,0.0933,0.0783,0.0963,0.1012,5.0866,0f000001,0*64f2f597\n\t", "INSPVAXA,USB3,0,51.0,FINESTEERING,2107,283539.100,02000000,471d,15824;INS_ALIGNMENT_COMPLETE,INS_RTKFIXED,37.37125716893,126.72240151116,7.9851,22.3000,0.0349,-0.3370,0.0409,-1.494089497,0.116619175,269.541070998,0.4422,0.2966,0.5733,0.1130,0.0931,0.0783,0.0963,0.1012,5.0845,0f000001,0*15f1df55\n\t", "INSPVAXA,USB3,0,51.0,FINESTEERING,2107,283539.600,02000000,471d,15824;INS_ALIGNMENT_COMPLETE,INS_RTKFIXED,37.37125727133,126.72239988665,7.9877,22.3000,0.0429,-0.2928,0.0329,-1.461817471,0.138335830,269.463131487,0.4422,0.2966,0.5733,0.1130,0.0931,0.0783,0.0963,0.1012,5.0845,0f000001,0*8c571713\n\t", "INSPVAXA,USB3,0,50.0,FINESTEERING,2107,283540.100,02000000,471d,15824;INS_ALIGNMENT_COMPLETE,INS_RTKFIXED,37.37125737761,126.72239824656,7.9900,22.3000,0.0519,-0.2782,0.0221,-1.451094613,0.074238516,269.298675528,0.4419,0.2969,0.5734,0.1130,0.0929,0.0783,0.0963,0.1012,5.0817,0f000001,0*b323d296\n\t", "INSPVAXA,USB3,0,50.0,FINESTEERING,2107,283540.600,02000000,471d,15824;INS_ALIGNMENT_COMPLETE,INS_RTKFIXED,37.37125746759,126.72239663487,7.9912,22.3000,0.0429,-0.2872,0.0160,-1.425165250,-0.019252695,269.086348976,0.4419,0.2969,0.5734,0.1130,0.0929,0.0783,0.0963,0.1012,5.0817,0f000001,0*88d26abe\n\t", "INSPVAXA,USB3,0,47.0,FINESTEERING,2107,283541.100,02000000,471d,15824;INS_ALIGNMENT_COMPLETE,INS_RTKFIXED,37.37125754334,126.72239500157,7.9927,22.3000,0.0440,-0.2830,0.0173,-1.652300860,-0.379493530,268.915877089,0.4417,0.2969,0.5736,0.1129,0.0927,0.0783,0.0963,0.1011,5.0789,0f000001,0*58806b1d\n\t", "INSPVAXA,USB3,0,47.0,FINESTEERING,2107,283541.600,02000000,471d,15824;INS_ALIGNMENT_COMPLETE,INS_RTKFIXED,37.37125761933,126.72239337708,7.9953,22.3000,0.0493,-0.2834,0.0162,-1.785773716,-0.511638678,268.665930676,0.4417,0.2969,0.5736,0.1129,0.0927,0.0783,0.0963,0.1011,5.0789,0f000001,0*bd9c5353\n\t", "INSPVAXA,USB3,0,48.5,FINESTEERING,2107,283542.100,02000000,471d,15824;INS_ALIGNMENT_COMPLETE,INS_RTKFIXED,37.37125769665,126.72239177679,7.9980,22.3000,0.0493,-0.2951,0.0235,-1.875048061,-0.540533252,268.386297576,0.4405,0.2966,0.5735,0.1128,0.0925,0.0783,0.0963,0.1011,5.0773,0f000001,0*2be40074\n\t", "INSPVAXA,USB3,0,48.5,FINESTEERING,2107,283542.600,02000000,471d,15824;INS_ALIGNMENT_COMPLETE,INS_RTKFIXED,37.37125775872,126.72239016301,7.9996,22.3000,0.0518,-0.3025,0.0218,-1.945640979,-0.365484318,268.174264778,0.4405,0.2966,0.5735,0.1128,0.0925,0.0783,0.0963,0.1011,5.0773,0f000001,0*896be2ff\n\t", "INSPVAXA,USB3,0,47.5,FINESTEERING,2107,283543.100,02000000,471d,15824;INS_ALIGNMENT_COMPLETE,INS_RTKFIXED,37.37125783022,126.72238854441,8.0007,22.3000,0.0360,-0.2808,0.0229,-1.906190638,-0.356725874,267.886535177,0.4398,0.2962,0.5735,0.1128,0.0925,0.0783,0.0963,0.1011,5.0772,0f000001,0*1744d296\n\t", "INSPVAXA,USB3,0,47.5,FINESTEERING,2107,283543.600,02000000,471d,15824;INS_ALIGNMENT_COMPLETE,INS_RTKFIXED,37.37125788763,126.72238692132,8.0016,22.3000,0.0356,-0.2896,0.0094,-1.979603347,-0.321373170,267.681718152,0.4398,0.2962,0.5735,0.1128,0.0925,0.0783,0.0963,0.1011,5.0772,0f000001,0*45f837fc\n\t", "DUALANTENNAHEADINGA,USB3,0,47.5,FINESTEERING,2107,283544.100,02000000,d426,15824;INSUFFICIENT_OBS,NONE,-1.000000000,0.000000000,0.000000000,0.0,0.000000000,0.000000000,\"631T\",12,4,4,3,04,00,20,02*84d96ce8\n\t", "INSPVAXA,USB3,0,51.0,FINESTEERING,2107,283544.600,02000000,471d,15824;INS_ALIGNMENT_COMPLETE,INS_RTKFIXED,37.37125797814,126.72238366933,8.0025,22.3000,0.0382,-0.2769,0.0143,-2.206615640,-0.357729210,267.363519498,0.4396,0.2961,0.5737,0.1128,0.0924,0.0783,0.0964,0.1011,5.0776,0f000001,0*0a578cde\n\t", "INSPVAXA,USB3,0,49.5,FINESTEERING,2107,283545.100,02000000,471d,15824;INS_ALIGNMENT_COMPLETE,INS_RTKFIXED,37.37125803132,126.72238203676,8.0019,22.3000,0.0517,-0.2764,0.0124,-2.158934023,-0.436592254,267.230007610,0.4389,0.2957,0.5737,0.1127,0.0924,0.0783,0.0964,0.1011,5.0787,0f000001,0*62787010\n\t", "INSPVAXA,USB3,0,49.5,FINESTEERING,2107,283545.600,02000000,471d,15824;INS_ALIGNMENT_COMPLETE,INS_RTKFIXED,37.37125808188,126.72238043700,8.0001,22.3000,0.0477,-0.2875,0.0096,-2.125628520,-0.371940065,267.210451376,0.4389,0.2957,0.5737,0.1127,0.0924,0.0783,0.0964,0.1011,5.0787,0f000001,0*6d8598a7\n\t", "DUALANTENNAHEADINGA,USB3,0,49.0,FINESTEERING,2107,283546.100,02000000,d426,15824;INSUFFICIENT_OBS,NONE,-1.000000000,0.000000000,0.000000000,0.0,0.000000000,0.000000000,\"631T\",14,4,4,3,04,00,20,03*f6e7f028\n\t", "INSPVAXA,USB3,0,49.0,FINESTEERING,2107,283546.600,02000000,471d,15824;INS_ALIGNMENT_COMPLETE,INS_RTKFIXED,37.37125815693,126.72237718708,7.9959,22.3000,0.0472,-0.2869,0.0097,-2.448876962,-0.301078601,267.272161666,0.4388,0.2955,0.5737,0.1127,0.0924,0.0783,0.0964,0.1011,5.0802,0f000001,0*b5ddd59b\n\t", "DUALANTENNAHEADINGA,USB3,0,49.0,FINESTEERING,2107,283547.100,02000000,d426,15824;INSUFFICIENT_OBS,NONE,-1.000000000,0.000000000,0.000000000,0.0,0.000000000,0.000000000,\"631T\",13,4,4,3,04,00,20,03*d1017fba\n\t", "DUALANTENNAHEADINGA,USB3,0,50.5,FINESTEERING,2107,283547.600,02000000,d426,15824;INSUFFICIENT_OBS,NONE,-1.000000000,0.000000000,0.000000000,0.0,0.000000000,0.000000000,\"631T\",14,4,4,3,04,00,20,03*23b2448a\n\t", "INSPVAXA,USB3,0,48.5,FINESTEERING,2107,283548.100,02000000,471d,15824;INS_ALIGNMENT_COMPLETE,INS_RTKFIXED,37.37125826747,126.72237261641,7.9908,22.3000,0.0551,-0.2062,0.0107,-2.709225073,-0.117327049,267.249046746,0.4386,0.2951,0.5737,0.1130,0.0926,0.0783,0.0964,0.1011,5.0831,0f000001,0*59a87063\n\t", "INSPVAXA,USB3,0,48.5,FINESTEERING,2107,283548.600,02000000,471d,15824;INS_ALIGNMENT_COMPLETE,INS_RTKFIXED,37.37125828182,126.72237093999,7.9873,22.3000,0.0467,-0.3123,0.0115,-2.842538161,-0.073425539,267.267184569,0.4386,0.2951,0.5737,0.1130,0.0926,0.0783,0.0964,0.1011,5.0831,0f000001,0*3db09e30\n\t", "INSPVAXA,USB3,0,49.0,FINESTEERING,2107,283549.100,02000000,471d,15824;INS_ALIGNMENT_COMPLETE,INS_RTKFIXED,37.37125831392,126.72236948257,7.9859,22.3000,0.0458,-0.3107,0.0117,-2.935659020,0.110600359,267.341322191,0.4389,0.2949,0.5737,0.1127,0.0927,0.0783,0.0964,0.1010,5.0837,0f000001,0*651f733f\n\t", "DUALANTENNAHEADINGA,USB3,0,49.0,FINESTEERING,2107,283549.600,02000000,d426,15824;INSUFFICIENT_OBS,NONE,-1.000000000,0.000000000,0.000000000,0.0,0.000000000,0.000000000,\"631T\",12,4,4,3,04,00,20,03*a5c8d3a9\n\t", "INSPVAXA,USB3,0,49.0,FINESTEERING,2107,283550.100,02000000,471d,15824;INS_ALIGNMENT_COMPLETE,INS_RTKFIXED,37.37125837980,126.72236622244,7.9865,22.3000,0.0464,-0.2979,0.0062,-2.970555166,0.308033741,267.553888887,0.4387,0.2947,0.5737,0.1126,0.0926,0.0783,0.0963,0.1010,5.0837,0f000001,0*d140be5a\n\t", "INSPVAXA,USB3,0,50.5,FINESTEERING,2107,283550.600,02000000,471d,15824;INS_ALIGNMENT_COMPLETE,INS_RTKFIXED,37.37125841199,126.72236465933,7.9851,22.3000,0.0388,-0.2917,0.0030,-2.826015531,0.302597414,267.642559027,0.4387,0.2947,0.5737,0.1126,0.0926,0.0783,0.0963,0.1010,5.0837,0f000001,0*d1068808\n\t", "DUALANTENNAHEADINGA,USB3,0,46.5,FINESTEERING,2107,283551.100,02000000,d426,15824;INSUFFICIENT_OBS,NONE,-1.000000000,0.000000000,0.000000000,0.0,0.000000000,0.000000000,\"631T\",12,4,4,3,04,00,20,03*69312952\n\t", "INSPVAXA,USB3,0,46.5,FINESTEERING,2107,283551.600,02000000,471d,15824;INS_ALIGNMENT_COMPLETE,INS_RTKFIXED,37.37125843948,126.72236147331,7.9829,22.3000,0.0386,-0.2728,0.0018,-2.861657525,0.138389194,267.863675039,0.4385,0.2948,0.5738,0.1126,0.0925,0.0783,0.0963,0.1010,5.0836,0f000001,0*5dcd711b\n\t", "DUALANTENNAHEADINGA,USB3,0,44.5,FINESTEERING,2107,283552.100,02000000,d426,15824;INSUFFICIENT_OBS,NONE,-1.000000000,0.000000000,0.000000000,0.0,0.000000000,0.000000000,\"631T\",13,4,4,3,04,00,20,03*c0320929\n\t", "DUALANTENNAHEADINGA,USB3,0,44.5,FINESTEERING,2107,283552.600,02000000,d426,15824;INSUFFICIENT_OBS,NONE,-1.000000000,0.000000000,0.000000000,0.0,0.000000000,0.000000000,\"631T\",14,4,4,3,04,00,20,03*46a498f4\n\t", "DUALANTENNAHEADINGA,USB3,0,44.5,FINESTEERING,2107,283553.100,02000000,d426,15824;INSUFFICIENT_OBS,NONE,-1.000000000,0.000000000,0.000000000,0.0,0.000000000,0.000000000,\"631T\",13,4,4,3,04,00,20,03*adea0df0\n\t", "INSPVAXA,USB3,0,48.5,FINESTEERING,2107,283553.600,02000000,471d,15824;INS_ALIGNMENT_COMPLETE,INS_RTKFIXED,37.37125846696,126.72235533990,7.9816,22.3000,0.0235,-0.2652,0.0170,-2.709628745,-0.144831569,268.295218513,0.4383,0.2948,0.5739,0.1125,0.0924,0.0783,0.0963,
